vi "TEST_PP_EventMarkers_Read.vi"() -> ()   [LabVIEW 2023]
uses:
  <vilib>/Rock Robotics/WPI/ThirdParty/MJansen/PathPlanner/PathPlanner24.lvlib
  <vilib>/Rock Robotics/WPI/ThirdParty/JAS_Junk/TrajLib/Trajectory_Library.lvlib
  <vilib>/Rock Robotics/WPI/ThirdParty/JAS_Junk/TrajLib/TypeDef/TRANSLATION2D.ctl
  <vilib>/Rock Robotics/WPI/ThirdParty/MJansen/PathPlanner/ENum/PathPlanner_CommandUtilType_ENUM.ctl
  <vilib>/Rock Robotics/WPI/ThirdParty/MJansen/PathPlanner/TypeDef/PathPlannerCommandUtil.ctl
  <vilib>/Rock Robotics/WPI/ThirdParty/MJansen/PathPlanner/TypeDef/PathPlannerEventMarker.ctl
panel:
  out "Timers":dbl[](array[numeric])
  out "Event Request":bool
  out "Event End":bool
  in  "FileName":string="C:\\Users\\Winston\\Documents\\LabVIEW Data\\FRC#8020 Swerve Drive Project 0201Y24\\deploy\\pathplanner\\paths\\Path_Testing_1.path"
  out "EventMarkers":T1[](array[typedef]) {"lastRobotPos"."Y" format="%14.3f"; "lastRobotPos"."X" format="%14.3f"; "markerPos"."Y" format="%14.3f"; "markerPos"."X" format="%14.3f"}
  out "error out":errorcluster
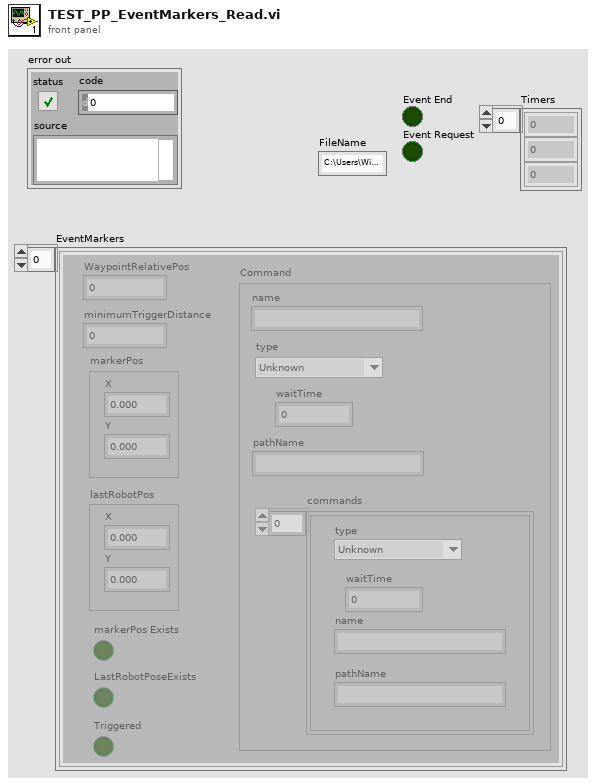
[diagram p1: front panel]
types:
  T1 = typedef "PathPlanner24.lvlib/PathPlannerEventMarker.ctl" = cluster{"WaypointRelativePos":dbl, "minimumTriggerDistance":dbl, "markerPos":T2, "lastRobotPos":T2, "Command":T3, "markerPos Exists":bool, "LastRobotPoseExists":bool, "Triggered":bool}
  T2 = typedef "Trajectory_Library.lvlib/TRANSLATION2D.ctl" = cluster{"X":dbl, "Y":dbl}
  T3 = typedef "PathPlanner24.lvlib/PathPlannerCommandUtil.ctl" = cluster{"waitTime":dbl, "name":string, "pathName":string, "commands":cluster{"type":T4, "waitTime":dbl, "name":string, "pathName":string}[], "type":T4}
  T4 = typedef "PathPlanner24.lvlib/PathPlanner_CommandUtilType_ENUM.ctl" = enum16{"Unknown", "Wait", "Named", "Path", "Sequential", "Parallel", "Race", "Deadline"}
  T5 = typedef "PathPlanner24.lvlib/PathPlannerPath.ctl" = cluster{"BezierPoints":T2[], "PreviewStartingRotation":T6, "Reversed":bool, "RotationTargets":T7[], "ConstraintZones":T8[], "EventMarkers":T1[], "GlobalConstraints":T9, "GoalEndState":T10, "AllPoints":T11[]}
  T6 = typedef "Trajectory_Library.lvlib/ROTATION2D.ctl" = cluster{"VALUE":dbl, "COS":dbl, "SIN":dbl}
  T7 = typedef "PathPlanner24.lvlib/PathPlannerRotationTarget.ctl" = cluster{"target":T6, "WaypointRelativePosition":dbl, "Exists":bool}
  T8 = typedef "PathPlanner24.lvlib/PathPlannerConstraintsZone.ctl" = cluster{"minWaypointPos":dbl, "maxWaypointPos":dbl, "Constraints":T9, "Present":bool}
  T9 = typedef "PathPlanner24.lvlib/PathPlannerPathConstraints.ctl" = cluster{"MaxVelocityMps;":dbl, "MaxAccelerationMpsSq;":dbl, "MaxAngularVelRadPsEc;":dbl, "MaxAngularAccRadPSecSq":dbl, "Exists":bool}
  T10 = typedef "PathPlanner24.lvlib/PathPlannerGoalEndState.ctl" = cluster{"Velocity":dbl, "Rotation":T6}
  T11 = typedef "PathPlanner24.lvlib/PathPlannerPathPoint.ctl" = cluster{"Position":T2, "HolonomicRotation":T6, "DistAlongPath":dbl, "CurveRadius":dbl, "MaxV":dbl, "Constraints":T9, "HolonomicRotationExists":bool}
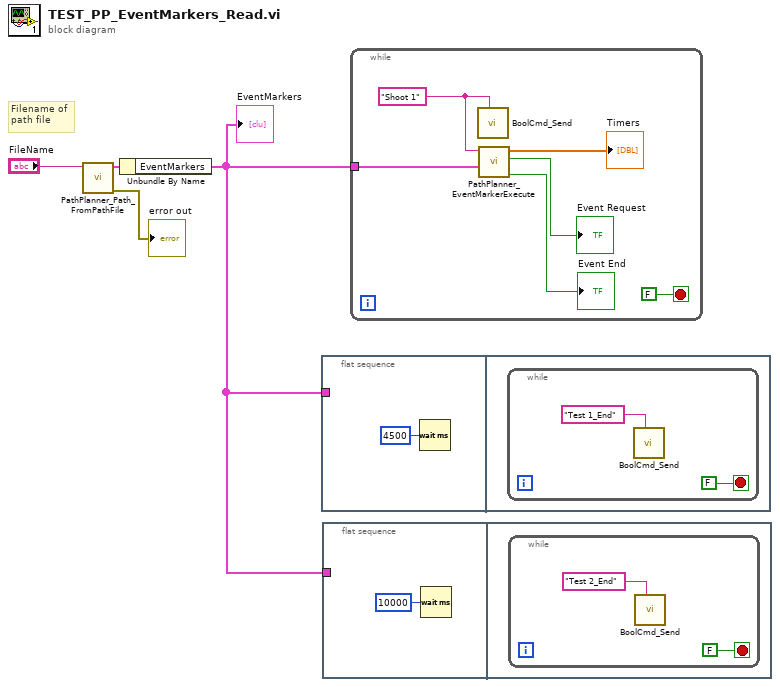
[diagram p0: block diagram]
diagram:
  # "Filename of\npath file"
  n1 = call <vilib>:"PathPlanner_Path_FromPathFile.vi"("FileName"="FileName") -> ("error out"=→"error out":errorcluster, "PathPlannerPath"=w2:T5)  [unwired: 8 in, 1 out]
  n2 = Unbundle By Name(w2) -> ("EventMarkers"=w1:T1[])
  "EventMarkers" <- w1
  n3 = flat-sequence {
    tunnel: w1 -> [_]
    frame #0 {
      n4 = Wait (ms)(milliseconds to wait=u32 4500) -> ()  [unwired: 1 out]
    }
    frame #1 {
      n5 = while {
        stop <- FALSE stop-if-true
        n6 = call <vilib>:"BoolCmd_Send.vi"("Command Name"="Test 1_End") -> ()  [unwired: 10 in, 1 out]
      }
    }
  }
  n7 = flat-sequence {
    tunnel: w1 -> [_]
    frame #0 {
      n8 = Wait (ms)(milliseconds to wait=u32 10000) -> ()  [unwired: 1 out]
    }
    frame #1 {
      n9 = while {
        stop <- FALSE stop-if-true
        n10 = call <vilib>:"BoolCmd_Send.vi"("Command Name"="Test 2_End") -> ()  [unwired: 10 in, 1 out]
      }
    }
  }
  n11 = while {
    tunnel: w1 -> [w11]
    stop <- FALSE stop-if-true
    w15 = "Shoot 1" ("Event Name")
    n12 = call <vilib>:"BoolCmd_Send.vi"("Command Name"=w15) -> ()  [unwired: 10 in, 1 out]
    n13 = call "PathPlanner_EventMarkerExecute.vi"("EventMarkers"=w11, "Event Name"=w15) -> ("Event End"=→"Event End":bool, "Event Request"=→"Event Request":bool, "Timers"=→"Timers":dbl[])  [unwired: 7 in]
  }
